vi "GetCountOf.vi"(8 "error in (no error)":errorcluster, 10 "Countable":variant) -> (0 "error out":errorcluster, 2 "Count":i32)   [LabVIEW 2019, in "Constraint.lvlib" / "Count.lvclass"]
uses:
  Count.lvclass
  <vilib>/Utility/error.llb/Error Cluster From Error Code.vi
  <vilib>/ErrorRing/Error Ring.xnode
  <vilib>/Utility/Data Type/Type Definitions/Data Type.ctl
  <vilib>/Utility/Data Type/NI_Data Type.lvlib
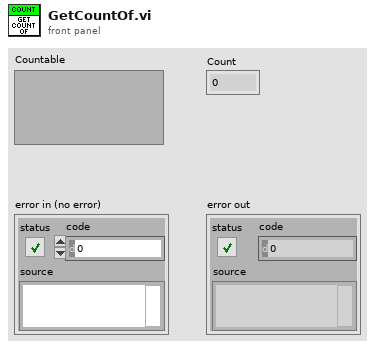
[diagram p1: front panel]
types:
  T1 = typedef "NI_Data Type.lvlib/Data Type.ctl" = enum8{"Invalid Type", "Void", "I8", "I16", "I32", "I64", "U8", "U16", "U32", "U64", "Single Float", "Double Float", "Extended Float", "Single Complex", "Double Complex", "Extended Complex", "Enum U8", "Enum U16", "Enum U32", "Enum U64", "Single Float With Unit", "Double Float With Unit", "Extended Float With Unit", "Single Complex with Unit", "Double Complex with Unit", "Extended Complex with Unit", "Boolean", "String", "Path", "Picture", "Tag", "Array", "Cluster", "Variant", "LV Variant", "Waveform", "Timestamp", "Digital Waveform", "Digital Data", "ExpressData", "Refnum", "External Data", "VI", "Poly VI", "LabVIEW Class Instance", "Fixed Point", "Set Collection", "Map Collection"}
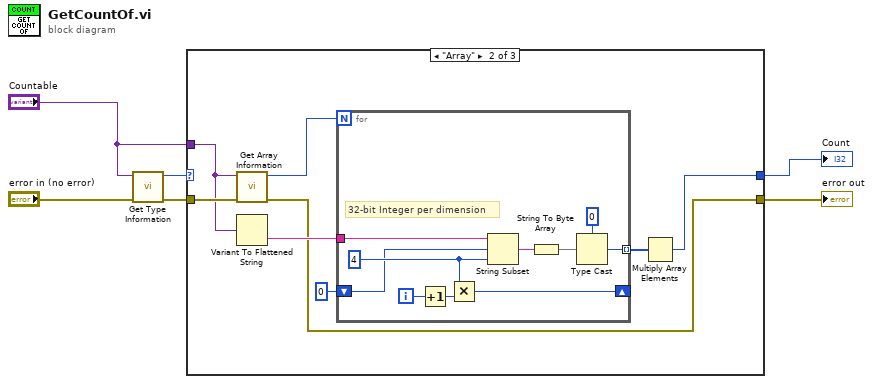
[diagram p0: block diagram]
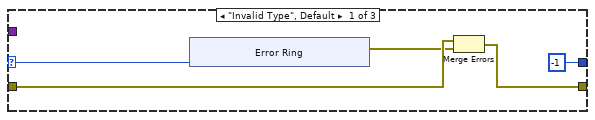
[diagram p2: hidden frame]
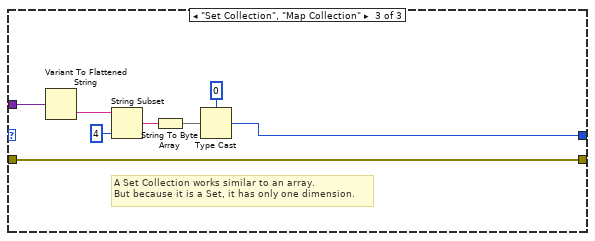
[diagram p3: hidden frame]
diagram:
  n1 = call <vilib>:"Get Type Information.vi"("error in (no error)"="error in (no error)", "variant"="Countable") -> ("error out"=w6:errorcluster, "type"=w5:T1)  [unwired: 5 in, 3 out]
  n2 = case shown="\"Array\"" w5 {
    selector: w5 -> [w9 _ _]
    tunnel: [-1 ("Count") w21 w38] -> w2
    tunnel: [w8 w22 w39] -> w1
    tunnel: w6 -> [w11 w26 w39]
    tunnel: "Countable" -> [_ w25 w41]
    frame "Invalid Type", Default {
      n3 = xnode "Error Ring"("parameter 0"=w9) -> ("error out"=w7:errorcluster)
      n4 = Merge Errors(w11, w7) -> (w8:errorcluster)
    }
    frame "Array" {
      n5 = call <vilib>:"Get Array Information.vi"("error in (no error)"=w26, "variant"=w25) -> ("error out"=w22:errorcluster, "number of dimensions"=w24:i32)  [unwired: 6 in, 2 out]
      n6 = Variant To Flattened String(Variant=w25) -> (data string=w23:string)  [unwired: 1 out]
      n7 = for {
        N: w24 -> [_]
        tunnel: w23 -> [w36]
        tunnel: [w29] -> w20 mode=indexing
        shift-right: [w33] -> _
        shift-left: 0 -> [w31]
        i -> [w34]
        w35 = 4 ("length (rest)")
        # "32-bit Integer per dimension"
        n8 = Increment(x=w34) -> (x+1=w32:i32)
        n9 = Multiply(x=w35, y=w32) -> (x*y=w33:i32)
        n10 = String Subset(string=w36, offset (0)=w31, length (rest)=w35) -> (substring=w30:string)
        n11 = String To Byte Array(string=w30) -> (unsigned byte array=w28:u8[])
        n12 = Type Cast(type=0, x=w28) -> (*(type *) &x=w29:i32)
      }
      n13 = Multiply Array Elements(1:w20) -> (0:w21:i32)
    }
    frame "Set Collection", "Map Collection" {
      # "A Set Collection works similar to an array.\nBut because it is a Set, it has only one dimension."
      n14 = Variant To Flattened String(Variant=w41) -> (data string=w40:string)  [unwired: 1 out]
      n15 = String Subset(string=w40, length (rest)=4 ("length (rest)")) -> (substring=w44:string)  [unwired: 1 in]
      n16 = String To Byte Array(string=w44) -> (unsigned byte array=w43:u8[])
      n17 = Type Cast(type=0, x=w43) -> (*(type *) &x=w38:i32)
    }
  }
  "error out" <- w1
  "Count" <- w2
